vi "GetSettingsRef.vi"(8 "error in (no error)":errorcluster, 11 "FpgaRef5761 in":refnum<class "FpgaRef5761.lvclass">) -> (0 "error out":errorcluster, 2 "Settings FPGA ref":T1, 3 "FpgaRef5761 out":refnum<class "FpgaRef5761.lvclass">)   [LabVIEW 2018, in "FpgaRef5761.lvclass"]
uses:
  FpgaRef5761.lvclass
  Scope/controls/settingsFPGAref.ctl
  FpgaRef5761.lvclass/FpgaRef5761.ctl
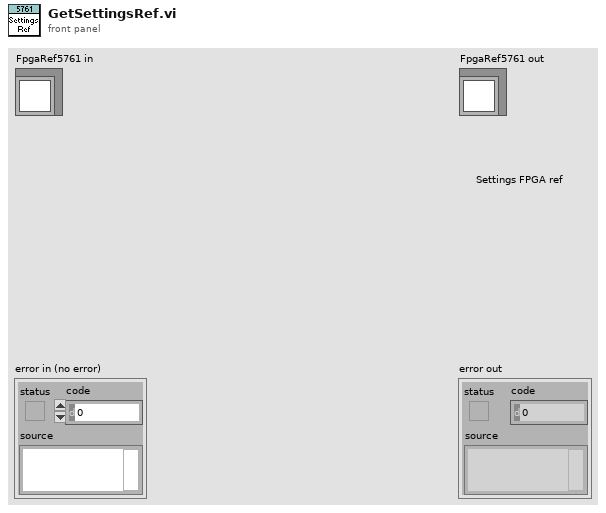
[diagram p1: front panel]
types:
  T1 = typedef "settingsFPGAref.ctl" = refnum<k20>
  T2 = typedef "5761 FPGA ref.ctl" = refnum<k20>
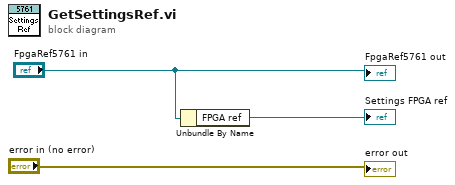
[diagram p0: block diagram]
diagram:
  n1 = Unbundle By Name("FpgaRef5761 in") -> ("FPGA ref"=→"Settings FPGA ref":T2)
  "error out" <- "error in (no error)"
  "FpgaRef5761 out" <- "FpgaRef5761 in"
